vi "Sequence.GenerateSequence.vi"(7 "Exists":bool, 8 "error in (no error)":errorcluster, 10 "Compiled Settings":T1, 11 "Path":path) -> (0 "error out":errorcluster)   [LabVIEW 2013, in "Simple Sequence Tools - Editor.lvlib"]
uses:
  Simple Sequence Tools - Editor.lvlib
  Types/Compiled.RTSequenceProperties.ctl
  Shared/Types/Channel.Properties.ctl
  Types/Compiled.StepProperties.ctl
  Types/Compiled.IOStateProperties.ctl
  Types/Compiled.StepElementProperties.ctl
  Shared/Types/Step.Types.ctl
  Types/Compiled.StepCondition.ctl
  Types/Conditions.OperationTypes.ctl
  Types/Compiled.SequenceChannels.ctl
  NationalInstruments.VeriStand.RealTimeSequenceDefinitionApi
  Shared/Simple Sequence Tools - Shared.lvlib
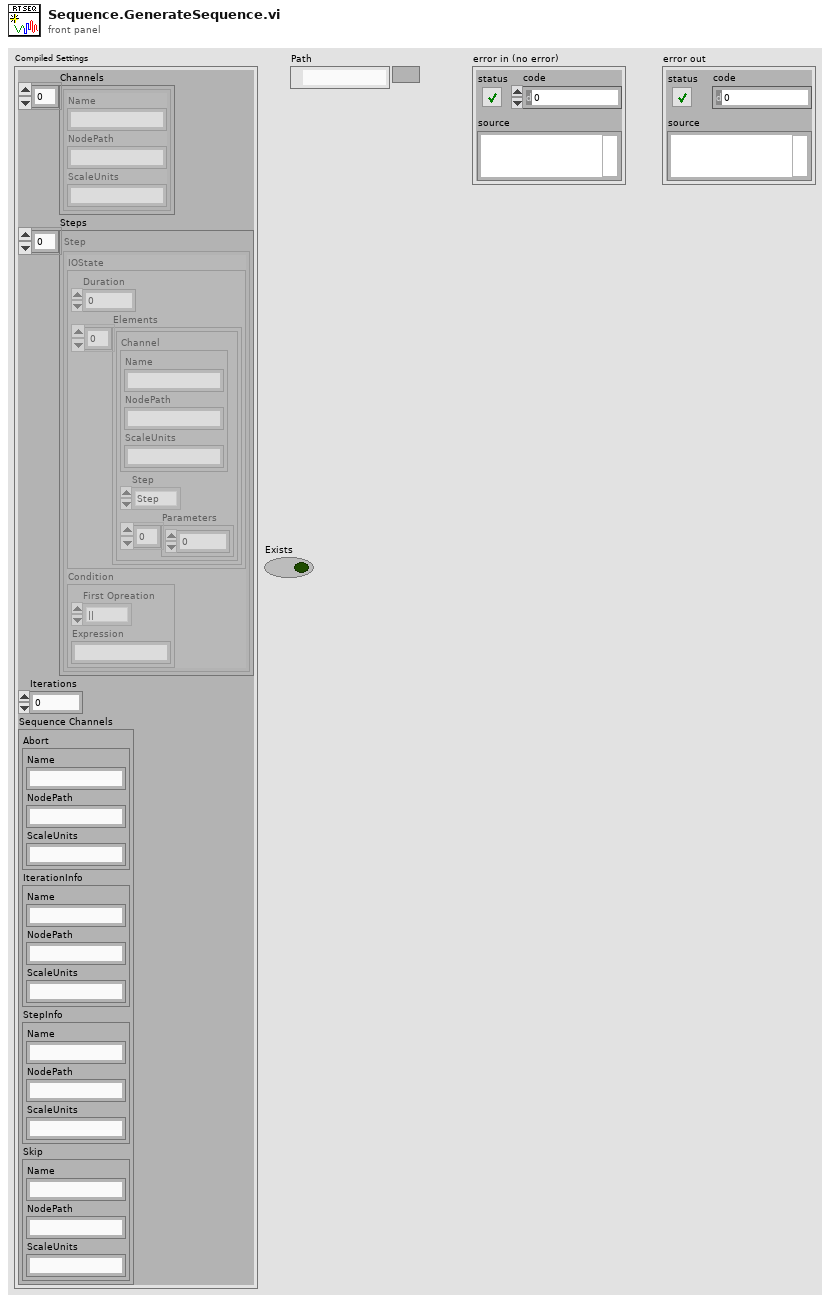
[diagram p1: front panel]
types:
  T1 = typedef "Simple Sequence Tools - Editor.lvlib/Compiled.RTSequenceProperties.ctl" = cluster{"Channels":T2[], "Steps":T3[], "Iterations":u32, "Sequence Channels":T9}
  T2 = typedef "Simple Sequence Tools - Shared.lvlib/Channel.Properties.ctl" = cluster{"Name":string, "NodePath":string, "ScaleUnits":string}
  T3 = typedef "Simple Sequence Tools - Editor.lvlib/Compiled.StepProperties.ctl" = cluster{"IOState":T4, "Condition":T7}
  T4 = typedef "Simple Sequence Tools - Editor.lvlib/Compiled.IOStateProperties.ctl" = cluster{"Duration":dbl, "Elements":T5[]}
  T5 = typedef "Simple Sequence Tools - Editor.lvlib/Compiled.StepElementProperties.ctl" = cluster{"Channel":T2, "Step":T6, "Parameters":dbl[]}
  T6 = typedef "Simple Sequence Tools - Shared.lvlib/Step.Types.ctl" = enum8{"Step", "iStep", "Ramp", "Unchanged", "Unknown", "Sine"}
  T7 = typedef "Simple Sequence Tools - Editor.lvlib/Compiled.StepCondition.ctl" = cluster{"First Opreation":T8, "Expression":string}
  T8 = typedef "Simple Sequence Tools - Editor.lvlib/Conditions.OperationTypes.ctl" = enum8{"None", "&&", "||"}
  T9 = typedef "Simple Sequence Tools - Editor.lvlib/Compiled.SequenceChannels.ctl" = cluster{"Abort":T2, "IterationInfo":T2, "StepInfo":T2, "Skip":T2}
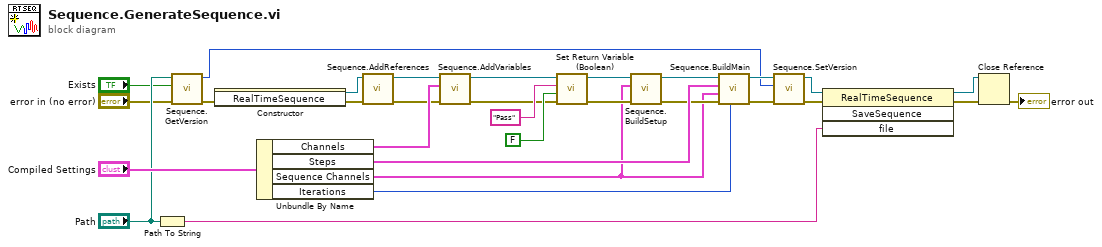
[diagram p0: block diagram]
diagram:
  n1 = Path To String(path="Path") -> (string=w21:string)
  n2 = call "Sequence.GetVersion.vi"("error in (no error)"="error in (no error)", "Exists"="Exists", "Path"="Path") -> ("error out"=w7:errorcluster, "Build"=w1:u32)  [unwired: 7 in]
  n3 = constructor class="RealTimeSequence"(error in=w7) -> (reference out=w20:refnum<k24>, error out=w12:errorcluster)  [unwired: 2 in, 1 out]
  n4 = Unbundle By Name("Compiled Settings") -> ("Channels"=w26:T2[], "Steps"=w17:T3[], "Sequence Channels"=w10:T9, "Iterations"=w11:u32)
  n5 = call "Sequence.AddReferences.vi"("error in (no error)"=w12, "Sequence"=w20) -> ("error out"=w18:errorcluster, "Sequence out"=w19:refnum<k24>)  [unwired: 8 in]
  n6 = call "Sequence.AddVariables.vi"("error in (no error)"=w18, "Channels"=w26, "Sequence"=w19) -> ("error out"=w25:errorcluster, "Sequence out"=w24:refnum<k24>)  [unwired: 7 in]
  n7 = call "Set Return Variable (Boolean).vi"("error in (no error)"=w25, "Value"=FALSE, "Identifier"="Pass", "Sequence Ref in"=w24) -> ("error out"=w16:errorcluster, "Sequence Ref out"=w15:refnum<k24>)  [unwired: 6 in]
  n8 = call "Sequence.BuildSetup.vi"("error in (no error)"=w16, "Sequence Channels"=w10, "Sequence"=w15) -> ("error out"=w13:errorcluster, "Sequence out"=w14:refnum<k24>)  [unwired: 7 in]
  n9 = call "Sequence.BuildMain.vi"("Iterations"=w11, "error in (no error)"=w13, "Sequence Channels"=w10, "Steps"=w17, "Sequence"=w14) -> ("error out"=w5:errorcluster, "Sequence out"=w3:refnum<k24>)  [unwired: 5 in]
  n10 = call "Sequence.SetVersion.vi"("error in (no error)"=w5, "BuildVersion"=w1, "RT Seq Ref"=w3) -> ("error out"=w4:errorcluster, "RT Seq Ref out"=w2:refnum<k24>)  [unwired: 7 in]
  n11 = invoke class="RealTimeSequence" method="SaveSequence"(reference=w2, error in=w4, "file"=w21) -> (reference out=w30:refnum<k24>, error out=w23:errorcluster)  [unwired: 1 in, 2 out]
  n12 = Close Reference(reference=w30, error in (no error)=w23) -> (error out=→"error out":errorcluster)
